vi "TestRun_Definitionen.vi"() -> (3 "Settings_Key_Ist_Soll":string[][](array[string]))   [LabVIEW 2020]
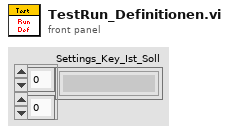
[diagram p1: front panel]
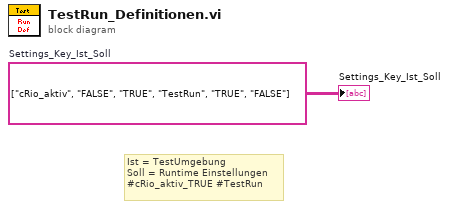
[diagram p0: block diagram]
diagram:
  w1 = string[][] [["cRio_aktiv", "FALSE", "TRUE"], ["TestRun", "TRUE", "FALSE"]]  # Settings_Key_Ist_Soll
  # "Ist = TestUmgebung\nSoll = Runtime Einstellungen\n#cRio_aktiv_TRUE #TestRun"
  "Settings_Key_Ist_Soll" <- w1
